vi "CheckSettings.vi"(0 "ChromaAcLoad in":refnum<class "ChromaAcLoad.lvclass">, 1 "RangeCheck":T1, 2 "Phase":i32, 3 "error in (no error)":errorcluster) -> (7 "ChromaAcLoad out":refnum<class "ChromaAcLoad.lvclass">, 10 "error out":errorcluster)   [LabVIEW 2018, in "AcPwrPlugins.lvlib" / "ChromaAcLoad.lvclass"]
doc: "This VI checks the value of the instrument settings and returns an error if the value is outside the instrument's range."
uses:
  ChromaAcLoad.lvclass
  TypeDefs/RangeCheck.ctl
  <vilib>/Utility/error.llb/Error Cluster From Error Code.vi
  <vilib>/ErrorRing/Error Ring.xnode
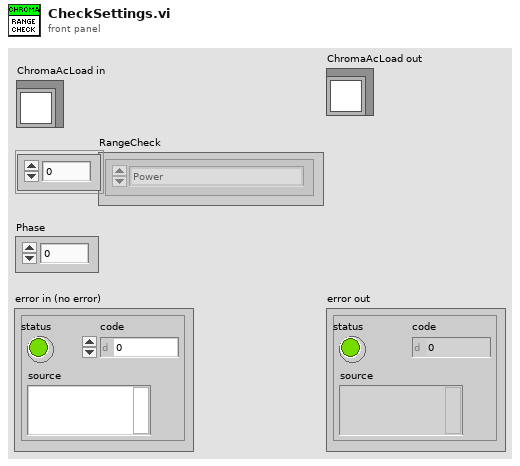
[diagram p1: front panel]
types:
  T1 = typedef "AcPwrPlugins.lvlib/ChromaAcLoad.lvclass/RangeCheck.ctl" = enum16{"Power", "Power Limit", "Current", "Current Peak", "Current Limit", "Voltage", "AC Resistance", "DC Resistance", "Frequency", "Crest Factor", "Power Factor", "RLC Power Factor", "Rise Slew Rate", "Fall Slew Rate", "Capacitance", "Inductance", "Parallel Resistance", "Series Resistance"}[]
  T2 = cluster{"Handle":string, "Name":string, "Phase Select":i32, "Instrument Options":string, "id query (T)":bool, "reset device (T)":bool, "Load Short Circuited":bool, "Line Synchronization":bool, "Load Current (A/Arms)":dbl, "Load Voltage (V/Vrms)":dbl, "Load Power (W)":dbl, "Load Resistance (Ohms)":dbl, "Load Current Peak Limit (A)":dbl, "Load Current Limit (A/Arms)":dbl, "Load Power Limit (W)":dbl, "Synch Frequency (Hz)":dbl, "Priority":enum16{"CF Only", "PF Only", "Both (CF)", "Both (PF)"}, "Crest Factor":dbl, "Power Factor":dbl, "Slew Rate":cluster{"Rise Slew Rate (A/ms)":i32, "Fall Slew Rate (A/ms)":i32}, "LC/RLC Mode":cluster{"Capacitance (uF)":i32, "Inductance (uH)":i32, "Series Resistance (Ohm)":dbl, "Parallel Resistance (Ohm)":dbl}, "Timing":cluster{"TimingOn":enum16{""}, "Hours":u32, "Minutes":u32, "Seconds":dbl, "CutoffVoltage":dbl}, "Connected":bool}[]
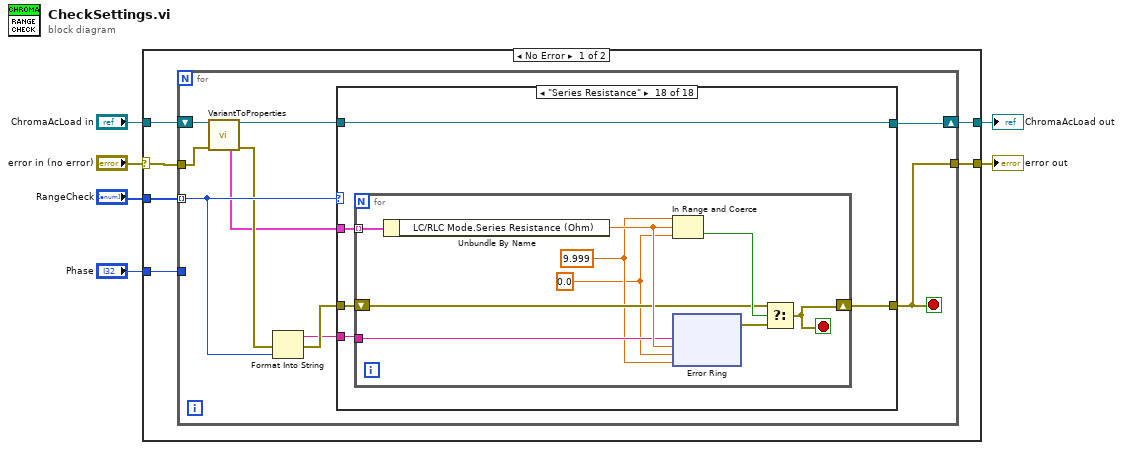
[diagram p0: block diagram]
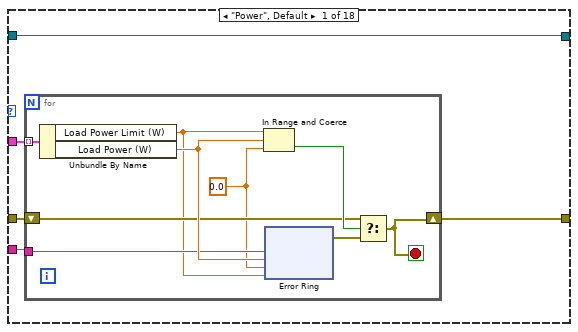
[diagram p2: hidden frame]
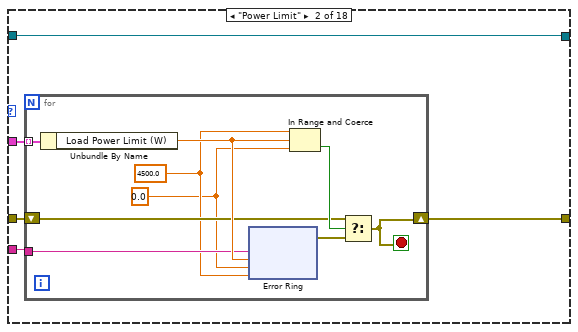
[diagram p3: hidden frame]
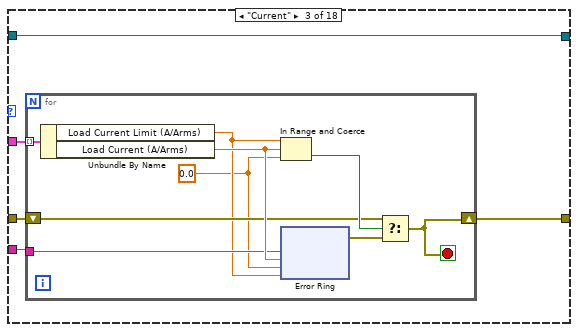
[diagram p4: hidden frame]
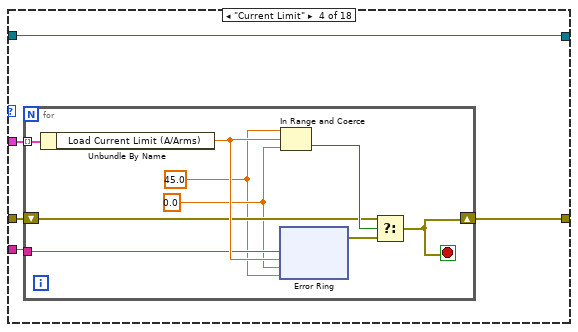
[diagram p5: hidden frame]
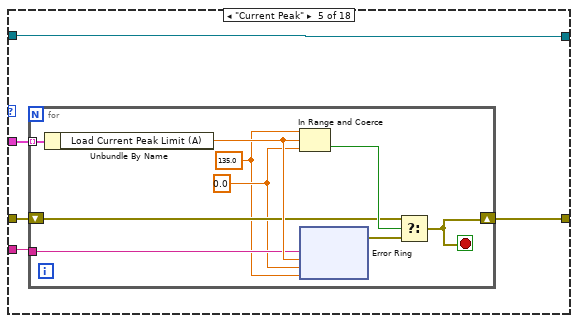
[diagram p6: hidden frame]
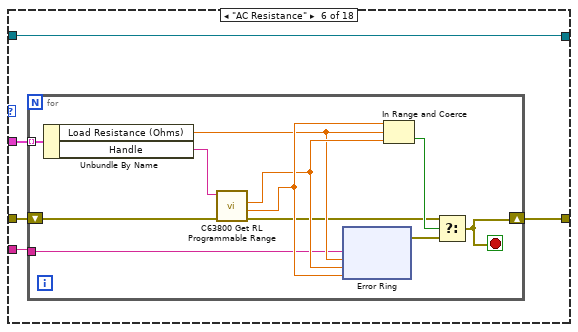
[diagram p7: hidden frame]
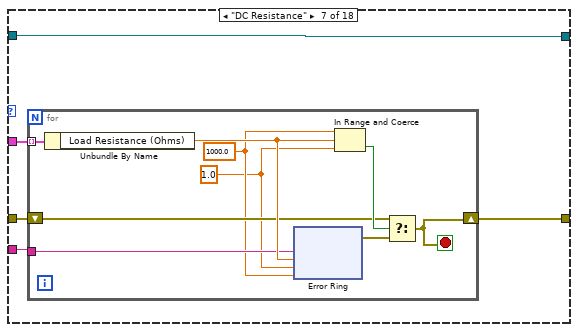
[diagram p8: hidden frame]
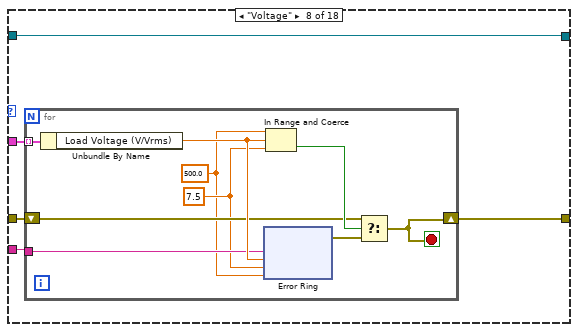
[diagram p9: hidden frame]
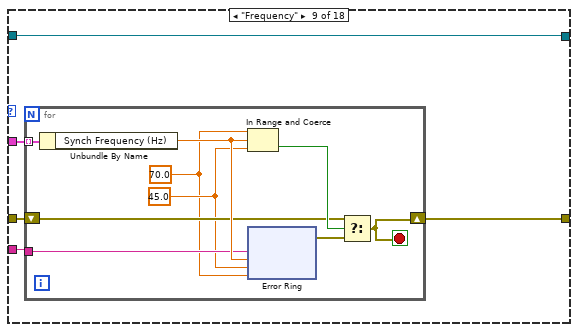
[diagram p10: hidden frame]
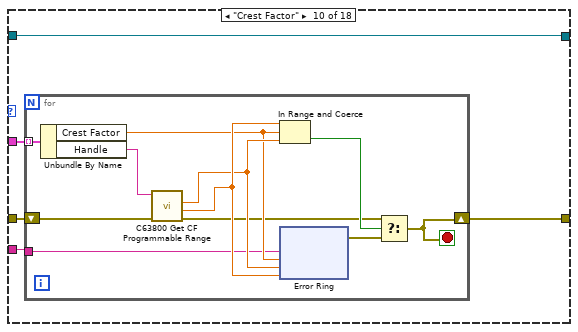
[diagram p11: hidden frame]
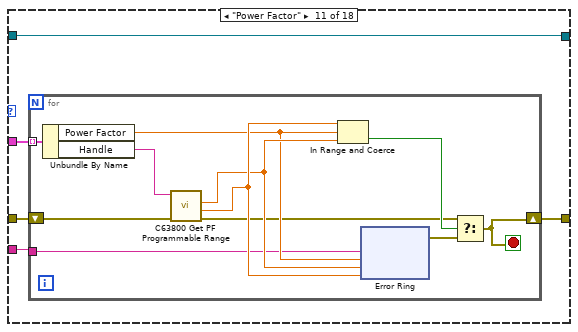
[diagram p12: hidden frame]
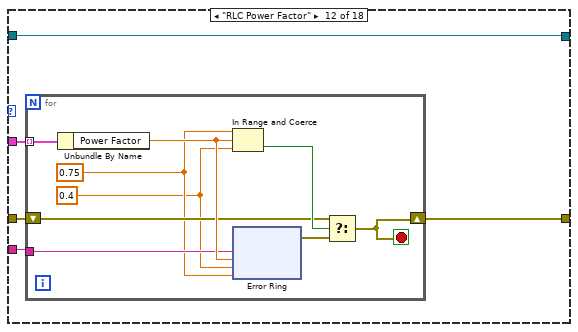
[diagram p13: hidden frame]
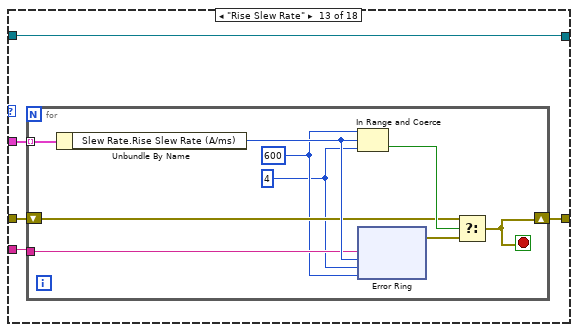
[diagram p14: hidden frame]
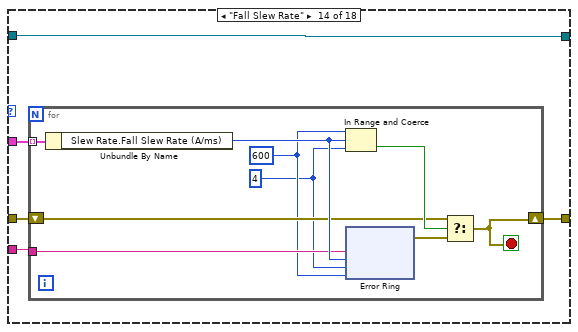
[diagram p15: hidden frame]
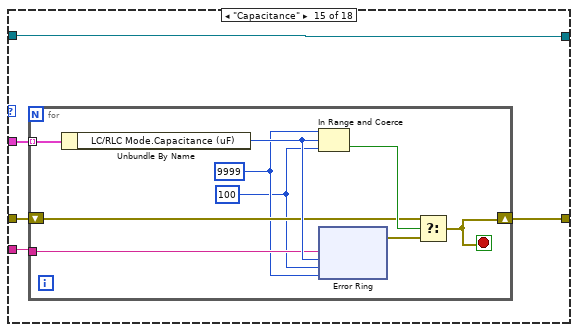
[diagram p16: hidden frame]
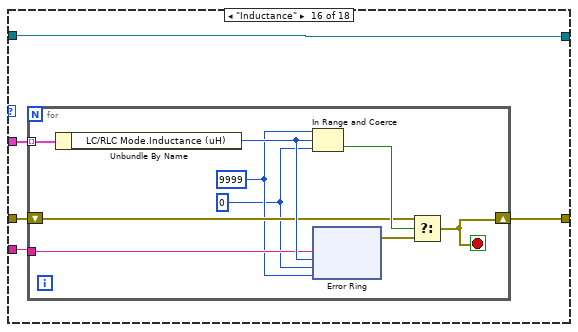
[diagram p17: hidden frame]
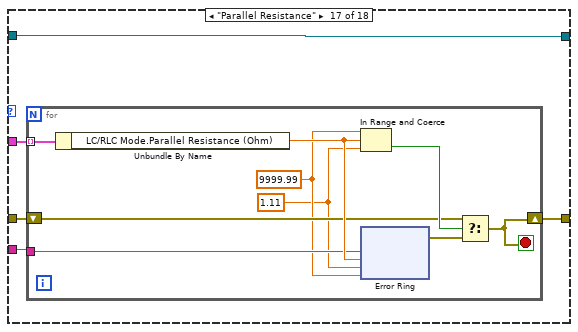
[diagram p18: hidden frame]
diagram:
  n1 = case shown="No Error" "error in (no error)" {
    selector: "error in (no error)" -> [w9 w461]
    tunnel: "ChromaAcLoad in" -> [w12 w462]
    tunnel: "Phase" -> [w11 _]
    tunnel: [w10 w462] -> w4
    tunnel: "RangeCheck" -> [w8 _]
    tunnel: [w7 w461] -> w1
    frame No Error {
      n2 = for {
        tunnel: w11 -> [_]
        shift-right: [w22] -> w10
        shift-left: w12 -> [w15]
        tunnel: w9 -> [w14]
        tunnel: w8 -> [w20] mode=indexing
        tunnel: [w21] -> w7
        stop <- w21 stop-if-true
        n3 = call "VariantToProperties.vi"("ChromaAcLoad"=w15, "error in (no error)"=w14) -> ("ChromaAcLoad"=w16:refnum<class "ChromaAcLoad.lvclass">, "Phases"=w13:T2, "error out"=w17:errorcluster)  [unwired: 7 in, 4 out]
        n4 = Format Into String(error in=w17, w20) -> (resulting string=w18:string, error out=w19:errorcluster)  [unwired: 2 in]
        n5 = case shown="\"Series Resistance\"" w20 {
          tunnel: w16 -> [w27 w51 w75 w99 w123 w147 w173 w197 w221 w245 w271 w297 w321 w345 w369 w393 w417 w441]
          tunnel: w19 -> [w23 w50 w74 w98 w122 w146 w172 w196 w220 w244 w270 w296 w320 w344 w368 w392 w416 w440]
          tunnel: [w27 w51 w75 w99 w123 w147 w173 w197 w221 w245 w271 w297 w321 w345 w369 w393 w417 w441] -> w22
          tunnel: [w26 w49 w73 w97 w121 w145 w171 w195 w219 w243 w269 w295 w319 w343 w367 w391 w415 w439] -> w21
          tunnel: w13 -> [w25 w48 w72 w95 w120 w144 w169 w193 w217 w241 w267 w293 w318 w342 w365 w390 w413 w437]
          tunnel: w18 -> [w24 w47 w71 w96 w119 w143 w170 w194 w218 w242 w268 w294 w317 w341 w366 w389 w414 w438]
          frame "Power", Default {
            n6 = for {
              shift-right: [w33] -> w26
              shift-left: w23 -> [w31]
              tunnel: w25 -> [w35] mode=indexing
              tunnel: w24 -> [w30]
              stop <- w33 stop-if-true
              w28 = 0.0 ("Load Power Limit (W)")
              n7 = Unbundle By Name(w35) -> ("Load Power Limit (W)"=w29:dbl, "Load Power (W)"=w32:dbl)
              n8 = In Range and Coerce(upper limit=w29, x=w32, lower limit=w28) -> (In Range?=w34:bool)  [unwired: 1 out]
              n9 = xnode "Error Ring"("parameter 0"=w30, "parameter 1"=w32, "parameter 2"=w28, "parameter 3"=w29) -> ("error out"=w36:errorcluster)
              n10 = Select(t=w31, s=w34, f=w36) -> (s? t:f=w33:errorcluster)
            }
          }
          frame "Power Limit" {
            n11 = for {
              shift-right: [w57] -> w49
              shift-left: w50 -> [w55]
              tunnel: w48 -> [w59] mode=indexing
              tunnel: w47 -> [w54]
              stop <- w57 stop-if-true
              w53 = 4500.0
              w52 = 0.0
              n12 = Unbundle By Name(w59) -> ("Load Power Limit (W)"=w56:dbl)
              n13 = xnode "Error Ring"("parameter 0"=w54, "parameter 1"=w56, "parameter 2"=w52, "parameter 3"=w53) -> ("error out"=w60:errorcluster)
              n14 = In Range and Coerce(upper limit=w53, x=w56, lower limit=w52) -> (In Range?=w58:bool)  [unwired: 1 out]
              n15 = Select(t=w55, s=w58, f=w60) -> (s? t:f=w57:errorcluster)
            }
          }
          frame "Current" {
            n16 = for {
              shift-right: [w81] -> w73
              shift-left: w74 -> [w79]
              tunnel: w72 -> [w83] mode=indexing
              tunnel: w71 -> [w78]
              stop <- w81 stop-if-true
              w76 = 0.0 ("Load Current (A/Arms)")
              n17 = Unbundle By Name(w83) -> ("Load Current Limit (A/Arms)"=w77:dbl, "Load Current (A/Arms)"=w80:dbl)
              n18 = In Range and Coerce(upper limit=w77, x=w80, lower limit=w76) -> (In Range?=w82:bool)  [unwired: 1 out]
              n19 = xnode "Error Ring"("parameter 0"=w78, "parameter 1"=w80, "parameter 2"=w76, "parameter 3"=w77) -> ("error out"=w84:errorcluster)
              n20 = Select(t=w79, s=w82, f=w84) -> (s? t:f=w81:errorcluster)
            }
          }
          frame "Current Limit" {
            n21 = for {
              shift-right: [w105] -> w97
              shift-left: w98 -> [w103]
              tunnel: w95 -> [w107] mode=indexing
              tunnel: w96 -> [w102]
              stop <- w105 stop-if-true
              w100 = 45.0
              w101 = 0.0
              n22 = Unbundle By Name(w107) -> ("Load Current Limit (A/Arms)"=w104:dbl)
              n23 = xnode "Error Ring"("parameter 0"=w102, "parameter 1"=w104, "parameter 2"=w101, "parameter 3"=w100) -> ("error out"=w108:errorcluster)
              n24 = In Range and Coerce(upper limit=w100, x=w104, lower limit=w101) -> (In Range?=w106:bool)  [unwired: 1 out]
              n25 = Select(t=w103, s=w106, f=w108) -> (s? t:f=w105:errorcluster)
            }
          }
          frame "Current Peak" {
            n26 = for {
              shift-right: [w129] -> w121
              shift-left: w122 -> [w127]
              tunnel: w120 -> [w131] mode=indexing
              tunnel: w119 -> [w126]
              stop <- w129 stop-if-true
              w124 = 135.0
              w125 = 0.0
              n27 = Unbundle By Name(w131) -> ("Load Current Peak Limit (A)"=w128:dbl)
              n28 = In Range and Coerce(upper limit=w124, x=w128, lower limit=w125) -> (In Range?=w130:bool)  [unwired: 1 out]
              n29 = xnode "Error Ring"("parameter 0"=w126, "parameter 1"=w128, "parameter 2"=w125, "parameter 3"=w124) -> ("error out"=w132:errorcluster)
              n30 = Select(t=w127, s=w130, f=w132) -> (s? t:f=w129:errorcluster)
            }
          }
          frame "AC Resistance" {
            n31 = for {
              shift-right: [w153] -> w145
              shift-left: w146 -> [w151]
              tunnel: w144 -> [w157] mode=indexing
              tunnel: w143 -> [w148]
              stop <- w153 stop-if-true
              n32 = Unbundle By Name(w157) -> ("Load Resistance (Ohms)"=w152:dbl, "Handle"=w149:string)
              n33 = call <instrlib>:"C63800 Get RL Programmable Range.vi"("error in (no error)"=w151, "Instrument Handle"=w149) -> ("error out"=w150:errorcluster, "Maximum"=w156:dbl, "Minimum"=w155:dbl)  [unwired: 6 in, 1 out]
              n34 = xnode "Error Ring"("parameter 0"=w148, "parameter 1"=w152, "parameter 2"=w155, "parameter 3"=w156) -> ("error out"=w158:errorcluster)
              n35 = In Range and Coerce(upper limit=w156, x=w152, lower limit=w155) -> (In Range?=w154:bool)  [unwired: 1 out]
              n36 = Select(t=w150, s=w154, f=w158) -> (s? t:f=w153:errorcluster)
            }
          }
          frame "DC Resistance" {
            n37 = for {
              shift-right: [w179] -> w171
              shift-left: w172 -> [w177]
              tunnel: w169 -> [w181] mode=indexing
              tunnel: w170 -> [w176]
              stop <- w179 stop-if-true
              w175 = 1000.0
              w174 = 1.0
              n38 = Unbundle By Name(w181) -> ("Load Resistance (Ohms)"=w178:dbl)
              n39 = xnode "Error Ring"("parameter 0"=w176, "parameter 1"=w178, "parameter 2"=w174, "parameter 3"=w175) -> ("error out"=w182:errorcluster)
              n40 = In Range and Coerce(upper limit=w175, x=w178, lower limit=w174) -> (In Range?=w180:bool)  [unwired: 1 out]
              n41 = Select(t=w177, s=w180, f=w182) -> (s? t:f=w179:errorcluster)
            }
          }
          frame "Voltage" {
            n42 = for {
              shift-right: [w203] -> w195
              shift-left: w196 -> [w201]
              tunnel: w193 -> [w205] mode=indexing
              tunnel: w194 -> [w200]
              stop <- w203 stop-if-true
              w198 = 500.0
              w199 = 7.5
              n43 = Unbundle By Name(w205) -> ("Load Voltage (V/Vrms)"=w202:dbl)
              n44 = xnode "Error Ring"("parameter 0"=w200, "parameter 1"=w202, "parameter 2"=w199, "parameter 3"=w198) -> ("error out"=w206:errorcluster)
              n45 = In Range and Coerce(upper limit=w198, x=w202, lower limit=w199) -> (In Range?=w204:bool)  [unwired: 1 out]
              n46 = Select(t=w201, s=w204, f=w206) -> (s? t:f=w203:errorcluster)
            }
          }
          frame "Frequency" {
            n47 = for {
              shift-right: [w227] -> w219
              shift-left: w220 -> [w225]
              tunnel: w217 -> [w229] mode=indexing
              tunnel: w218 -> [w224]
              stop <- w227 stop-if-true
              w222 = 70.0 ("Minimum")
              w223 = 45.0 ("Minimum")
              n48 = Unbundle By Name(w229) -> ("Synch Frequency (Hz)"=w226:dbl)
              n49 = In Range and Coerce(upper limit=w222, x=w226, lower limit=w223) -> (In Range?=w228:bool)  [unwired: 1 out]
              n50 = xnode "Error Ring"("parameter 0"=w224, "parameter 1"=w226, "parameter 2"=w223, "parameter 3"=w222) -> ("error out"=w230:errorcluster)
              n51 = Select(t=w225, s=w228, f=w230) -> (s? t:f=w227:errorcluster)
            }
          }
          frame "Crest Factor" {
            n52 = for {
              shift-right: [w251] -> w243
              shift-left: w244 -> [w249]
              tunnel: w241 -> [w255] mode=indexing
              tunnel: w242 -> [w246]
              stop <- w251 stop-if-true
              n53 = Unbundle By Name(w255) -> ("Crest Factor"=w250:dbl, "Handle"=w247:string)
              n54 = call <instrlib>:"C63800 Get CF Programmable Range.vi"("error in (no error)"=w249, "Instrument Handle"=w247) -> ("error out"=w248:errorcluster, "Maximum"=w254:dbl, "Minimum"=w253:dbl)  [unwired: 6 in, 1 out]
              n55 = In Range and Coerce(upper limit=w254, x=w250, lower limit=w253) -> (In Range?=w252:bool)  [unwired: 1 out]
              n56 = xnode "Error Ring"("parameter 0"=w246, "parameter 1"=w250, "parameter 2"=w253, "parameter 3"=w254) -> ("error out"=w256:errorcluster)
              n57 = Select(t=w248, s=w252, f=w256) -> (s? t:f=w251:errorcluster)
            }
          }
          frame "Power Factor" {
            n58 = for {
              shift-right: [w277] -> w269
              shift-left: w270 -> [w275]
              tunnel: w267 -> [w281] mode=indexing
              tunnel: w268 -> [w272]
              stop <- w277 stop-if-true
              n59 = Unbundle By Name(w281) -> ("Power Factor"=w276:dbl, "Handle"=w273:string)
              n60 = call <instrlib>:"C63800 Get PF Programmable Range.vi"("error in (no error)"=w275, "Instrument Handle"=w273) -> ("error out"=w274:errorcluster, "Maximum"=w280:dbl, "Minimum"=w279:dbl)  [unwired: 6 in, 1 out]
              n61 = In Range and Coerce(upper limit=w280, x=w276, lower limit=w279) -> (In Range?=w278:bool)  [unwired: 1 out]
              n62 = xnode "Error Ring"("parameter 0"=w272, "parameter 1"=w276, "parameter 2"=w279, "parameter 3"=w280) -> ("error out"=w282:errorcluster)
              n63 = Select(t=w274, s=w278, f=w282) -> (s? t:f=w277:errorcluster)
            }
          }
          frame "RLC Power Factor" {
            n64 = for {
              shift-right: [w303] -> w295
              shift-left: w296 -> [w301]
              tunnel: w293 -> [w305] mode=indexing
              tunnel: w294 -> [w300]
              stop <- w303 stop-if-true
              w299 = 0.75
              w298 = 0.4
              n65 = Unbundle By Name(w305) -> ("Power Factor"=w302:dbl)
              n66 = In Range and Coerce(upper limit=w299, x=w302, lower limit=w298) -> (In Range?=w304:bool)  [unwired: 1 out]
              n67 = xnode "Error Ring"("parameter 0"=w300, "parameter 1"=w302, "parameter 2"=w298, "parameter 3"=w299) -> ("error out"=w306:errorcluster)
              n68 = Select(t=w301, s=w304, f=w306) -> (s? t:f=w303:errorcluster)
            }
          }
          frame "Rise Slew Rate" {
            n69 = for {
              shift-right: [w327] -> w319
              shift-left: w320 -> [w325]
              tunnel: w318 -> [w329] mode=indexing
              tunnel: w317 -> [w324]
              stop <- w327 stop-if-true
              w323 = 600
              w322 = 4
              n70 = Unbundle By Name(w329) -> ("Slew Rate.Rise Slew Rate (A/ms)"=w326:i32)
              n71 = In Range and Coerce(upper limit=w323, x=w326, lower limit=w322) -> (In Range?=w328:bool)  [unwired: 1 out]
              n72 = xnode "Error Ring"("parameter 0"=w324, "parameter 1"=w326, "parameter 2"=w322, "parameter 3"=w323) -> ("error out"=w330:errorcluster)
              n73 = Select(t=w325, s=w328, f=w330) -> (s? t:f=w327:errorcluster)
            }
          }
          frame "Fall Slew Rate" {
            n74 = for {
              shift-right: [w351] -> w343
              shift-left: w344 -> [w349]
              tunnel: w342 -> [w353] mode=indexing
              tunnel: w341 -> [w348]
              stop <- w351 stop-if-true
              w347 = 600
              w346 = 4
              n75 = Unbundle By Name(w353) -> ("Slew Rate.Fall Slew Rate (A/ms)"=w350:i32)
              n76 = In Range and Coerce(upper limit=w347, x=w350, lower limit=w346) -> (In Range?=w352:bool)  [unwired: 1 out]
              n77 = xnode "Error Ring"("parameter 0"=w348, "parameter 1"=w350, "parameter 2"=w346, "parameter 3"=w347) -> ("error out"=w354:errorcluster)
              n78 = Select(t=w349, s=w352, f=w354) -> (s? t:f=w351:errorcluster)
            }
          }
          frame "Capacitance" {
            n79 = for {
              shift-right: [w375] -> w367
              shift-left: w368 -> [w373]
              tunnel: w365 -> [w377] mode=indexing
              tunnel: w366 -> [w372]
              stop <- w375 stop-if-true
              w371 = 9999
              w370 = 100
              n80 = Unbundle By Name(w377) -> ("LC/RLC Mode.Capacitance (uF)"=w374:i32)
              n81 = In Range and Coerce(upper limit=w371, x=w374, lower limit=w370) -> (In Range?=w376:bool)  [unwired: 1 out]
              n82 = xnode "Error Ring"("parameter 0"=w372, "parameter 1"=w374, "parameter 2"=w370, "parameter 3"=w371) -> ("error out"=w378:errorcluster)
              n83 = Select(t=w373, s=w376, f=w378) -> (s? t:f=w375:errorcluster)
            }
          }
          frame "Inductance" {
            n84 = for {
              shift-right: [w399] -> w391
              shift-left: w392 -> [w397]
              tunnel: w390 -> [w401] mode=indexing
              tunnel: w389 -> [w396]
              stop <- w399 stop-if-true
              w395 = 9999
              w394 = 0
              n85 = Unbundle By Name(w401) -> ("LC/RLC Mode.Inductance (uH)"=w398:i32)
              n86 = In Range and Coerce(upper limit=w395, x=w398, lower limit=w394) -> (In Range?=w400:bool)  [unwired: 1 out]
              n87 = xnode "Error Ring"("parameter 0"=w396, "parameter 1"=w398, "parameter 2"=w394, "parameter 3"=w395) -> ("error out"=w402:errorcluster)
              n88 = Select(t=w397, s=w400, f=w402) -> (s? t:f=w399:errorcluster)
            }
          }
          frame "Parallel Resistance" {
            n89 = for {
              shift-right: [w423] -> w415
              shift-left: w416 -> [w421]
              tunnel: w413 -> [w425] mode=indexing
              tunnel: w414 -> [w420]
              stop <- w423 stop-if-true
              w419 = 9999.99
              w418 = 1.11
              n90 = Unbundle By Name(w425) -> ("LC/RLC Mode.Parallel Resistance (Ohm)"=w422:dbl)
              n91 = In Range and Coerce(upper limit=w419, x=w422, lower limit=w418) -> (In Range?=w424:bool)  [unwired: 1 out]
              n92 = xnode "Error Ring"("parameter 0"=w420, "parameter 1"=w422, "parameter 2"=w418, "parameter 3"=w419) -> ("error out"=w426:errorcluster)
              n93 = Select(t=w421, s=w424, f=w426) -> (s? t:f=w423:errorcluster)
            }
          }
          frame "Series Resistance" {
            n94 = for {
              shift-right: [w447] -> w439
              shift-left: w440 -> [w445]
              tunnel: w437 -> [w449] mode=indexing
              tunnel: w438 -> [w444]
              stop <- w447 stop-if-true
              w443 = 9.999
              w442 = 0.0
              n95 = Unbundle By Name(w449) -> ("LC/RLC Mode.Series Resistance (Ohm)"=w446:dbl)
              n96 = In Range and Coerce(upper limit=w443, x=w446, lower limit=w442) -> (In Range?=w448:bool)  [unwired: 1 out]
              n97 = xnode "Error Ring"("parameter 0"=w444, "parameter 1"=w446, "parameter 2"=w442, "parameter 3"=w443) -> ("error out"=w450:errorcluster)
              n98 = Select(t=w445, s=w448, f=w450) -> (s? t:f=w447:errorcluster)
            }
          }
        }
      }
    }
    frame Error {
    }
  }
  "error out" <- w1
  "ChromaAcLoad out" <- w4
